vi "HWCEventHandler.vi"(8 "error in (no error)":errorcluster, 11 "HWController in":refnum<class "HWController.lvclass">) -> (0 "error out":errorcluster, 3 "HWController out":refnum<class "HWController.lvclass">)   [LabVIEW 2009, in "Hardware.lvlib" / "HWControllers.lvlib" / "HWController.lvclass"]
uses:
  HWController.lvclass
  HWController.lvclass/HWController.ctl
  HWControllerEvents/HWControllerEvents.lvclass
panel:
  out "configureTime":dbl
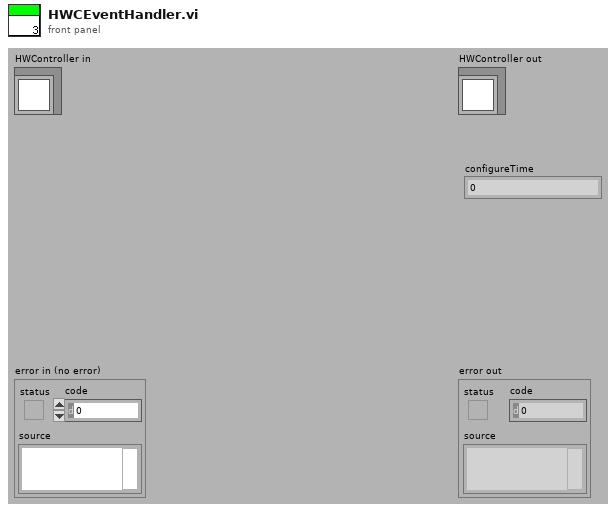
[diagram p1: front panel]
types:
  T1 = enum16{"Ready", "Compiling", "Configured", "Running", "Stopping", "Unresolved Error"}
  T2 = cluster{"incomingEventTypes":cluster{"start":cluster{"Boolean":bool}, "stop":cluster{"Boolean":bool}, "statusInquiry":cluster{"Boolean":bool}, "configure":cluster{"DPScriptPath":path, "TimeStamp":string, "HWLoop?":bool}, "resetError":cluster{"Boolean":bool}, "resourcesInquiry":cluster{"Boolean":bool}, "reserveResources":cluster{"HWList":string[]}, "initialise":cluster{"HWList":string[]}, "close":cluster{"Boolean":bool}, "resetAllChannels":cluster{"Boolean":bool}, "staticChannelUpdate":cluster{"channel_address":string, "calibratedValue":dbl}, "runScript":cluster{"DPScriptPath":path, "TimeStamp":string, "HWLoop?":bool}, "compilingScript":cluster{"Path":path}, "compiledScript":cluster{"Path":path, "timeCompileAt":string}, "compilerError":cluster{"Path":path}, "configureCompiledScript":cluster{"DPScriptPath":path, "TimeStamp":string, "HWLoop?":bool, "CompiledScript":cluster{"ScriptListCompiler.lvclass":refnum<class "ScriptListCompiler.lvclass">, "aoChannels":refnum<class "AnalogOutput.lvclass">[], "doChannels":refnum<class "DigitalOutput.lvclass">[], "rfChannels":refnum<class "DDSOutput.lvclass">[]}}, "restartCompiler":cluster{"restart":bool}, "staticRfChannelUpdate":cluster{"channel_address":string, "Output":cluster{"Frequency(MHz)":dbl, "Amplitude":dbl, "Phase":dbl, "OutputForm":enum16{"Sine", "Square", "Triangle", "Arbitrary"}}}}, "outgoingEventTypes":cluster{"HWStatus":cluster{"status":enum16{"Ready", "Compiling", "Configured", "Running", "Stopping", "Unresolved Error"}}, "error":cluster{"error out":errorcluster}, "resourcesAvailable":cluster{"availableHWList":string[], "reservedHWList":string[]}, "resourcesReserved":cluster{"reservedHWList":string[]}}}
  T3 = enum16{"start", "stop", "statusInquiry", "configure", "resetError", "resourcesInquiry", "reserveResources", "initialise", "resetAllChannels", "staticUpdate", "close", "HWStatus", "error", "resourcesAvailable", "resourcesReserved", "compilerError", "compiledScript", "compilingScript", "runScript", "configureCompiledScript", "restartCompiler", "staticRfChannelUpdate"}
  T4 = cluster{"start":cluster{"Boolean":bool}, "stop":cluster{"Boolean":bool}, "statusInquiry":cluster{"Boolean":bool}, "configure":cluster{"DPScriptPath":path, "TimeStamp":string, "HWLoop?":bool}, "resetError":cluster{"Boolean":bool}, "resourcesInquiry":cluster{"Boolean":bool}, "reserveResources":cluster{"HWList":string[]}, "initialise":cluster{"HWList":string[]}, "close":cluster{"Boolean":bool}, "resetAllChannels":cluster{"Boolean":bool}, "staticChannelUpdate":cluster{"channel_address":string, "calibratedValue":dbl}, "runScript":cluster{"DPScriptPath":path, "TimeStamp":string, "HWLoop?":bool}, "compilingScript":cluster{"Path":path}, "compiledScript":cluster{"Path":path, "timeCompileAt":string}, "compilerError":cluster{"Path":path}, "configureCompiledScript":cluster{"DPScriptPath":path, "TimeStamp":string, "HWLoop?":bool, "CompiledScript":cluster{"ScriptListCompiler.lvclass":refnum<class "ScriptListCompiler.lvclass">, "aoChannels":refnum<class "AnalogOutput.lvclass">[], "doChannels":refnum<class "DigitalOutput.lvclass">[], "rfChannels":refnum<class "DDSOutput.lvclass">[]}}, "restartCompiler":cluster{"restart":bool}, "staticRfChannelUpdate":cluster{"channel_address":string, "Output":cluster{"Frequency(MHz)":dbl, "Amplitude":dbl, "Phase":dbl, "OutputForm":enum16{"Sine", "Square", "Triangle", "Arbitrary"}}}}
  T5 = cluster{"DPScriptPath":path, "TimeStamp":string, "HWLoop?":bool}
  T6 = cluster{"DPScriptPath":path, "TimeStamp":string, "HWLoop?":bool, "CompiledScript":cluster{"ScriptListCompiler.lvclass":refnum<class "ScriptListCompiler.lvclass">, "aoChannels":refnum<class "AnalogOutput.lvclass">[], "doChannels":refnum<class "DigitalOutput.lvclass">[], "rfChannels":refnum<class "DDSOutput.lvclass">[]}}
  T7 = cluster{"ScriptListCompiler.lvclass":refnum<class "ScriptListCompiler.lvclass">, "aoChannels":refnum<class "AnalogOutput.lvclass">[], "doChannels":refnum<class "DigitalOutput.lvclass">[], "rfChannels":refnum<class "DDSOutput.lvclass">[]}
  T8 = cluster{"channel_address":string, "calibratedValue":dbl}
  T9 = cluster{"channel_address":string, "Output":cluster{"Frequency(MHz)":dbl, "Amplitude":dbl, "Phase":dbl, "OutputForm":enum16{"Sine", "Square", "Triangle", "Arbitrary"}}}
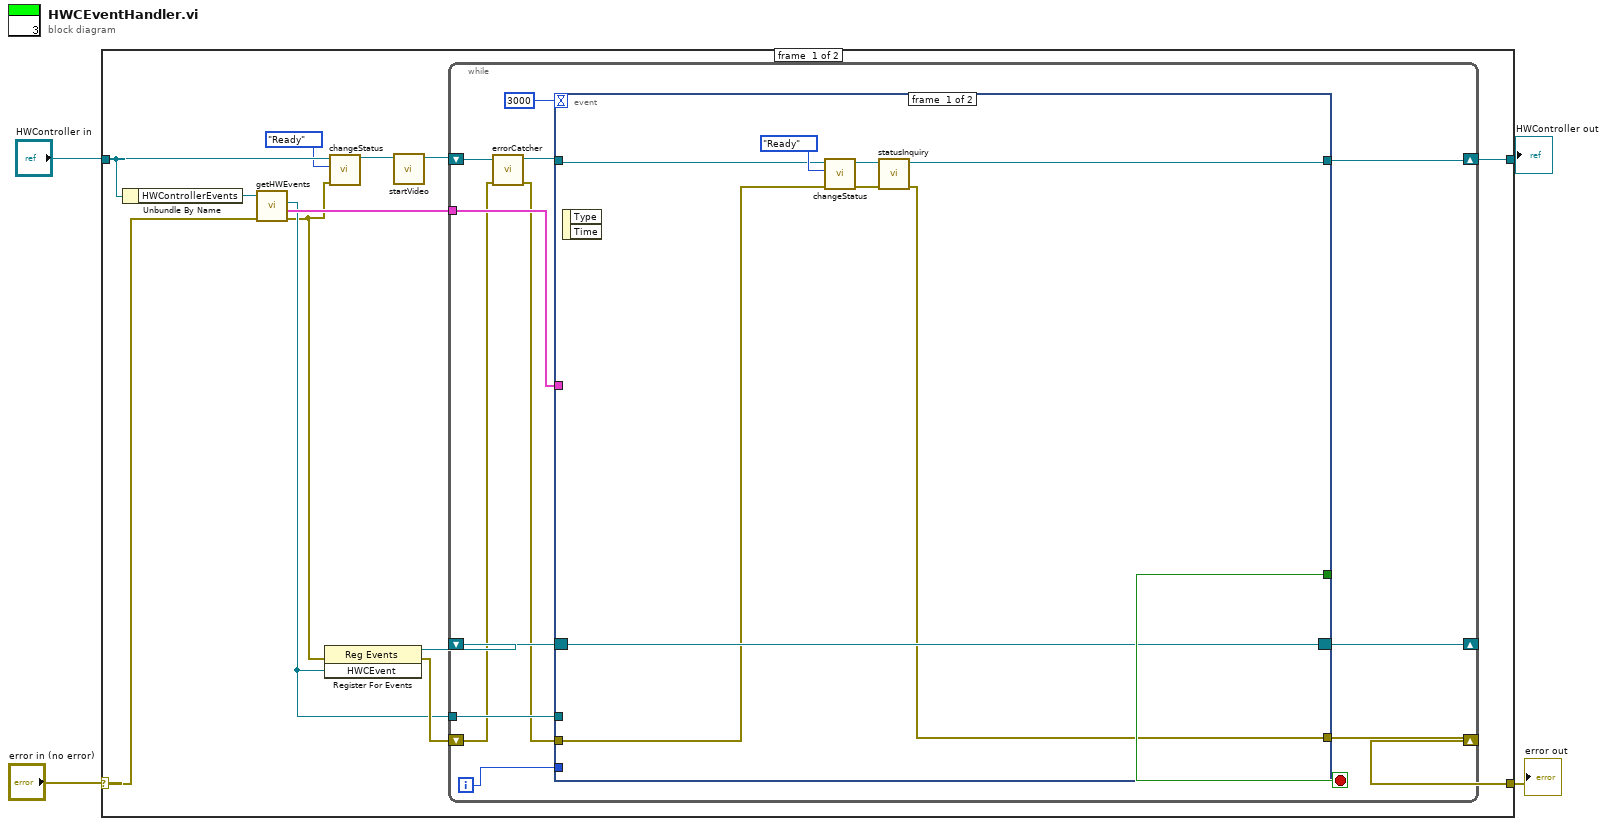
[diagram p0: block diagram]
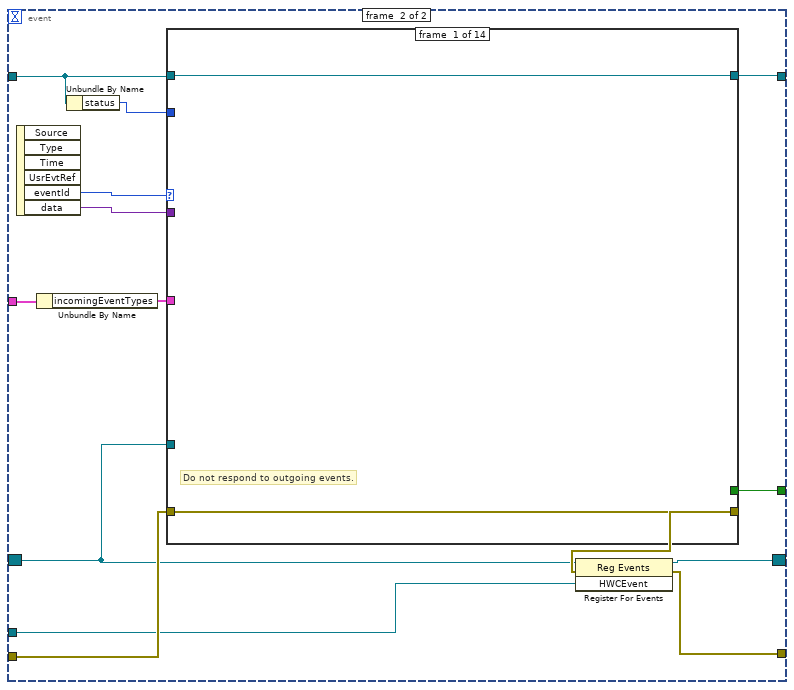
[diagram p2: hidden frame]
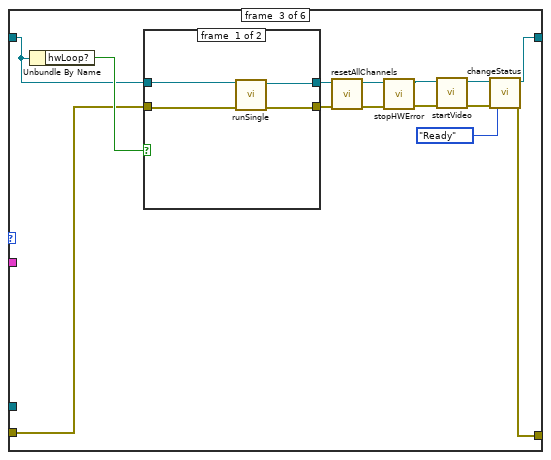
[diagram p5: hidden frame]
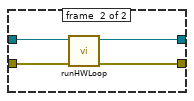
[diagram p6: hidden frame]
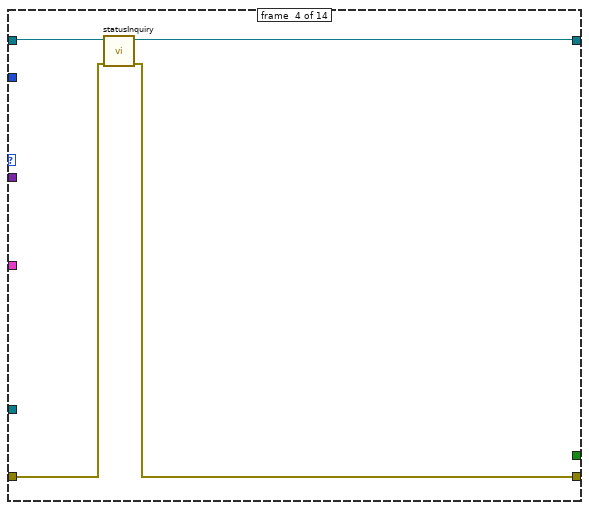
[diagram p11: hidden frame]
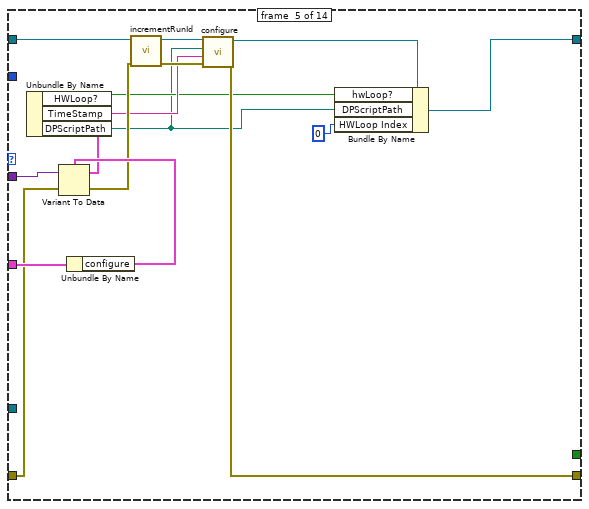
[diagram p12: hidden frame]
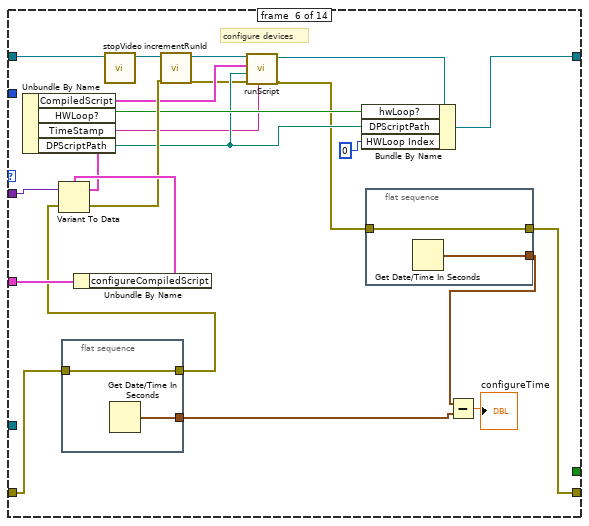
[diagram p13: hidden frame]
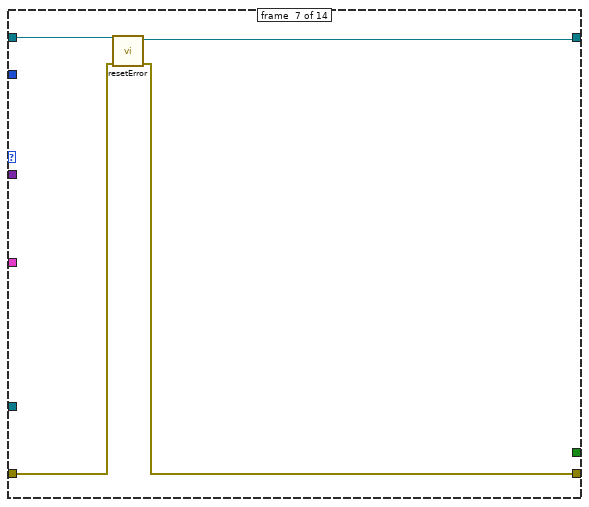
[diagram p14: hidden frame]
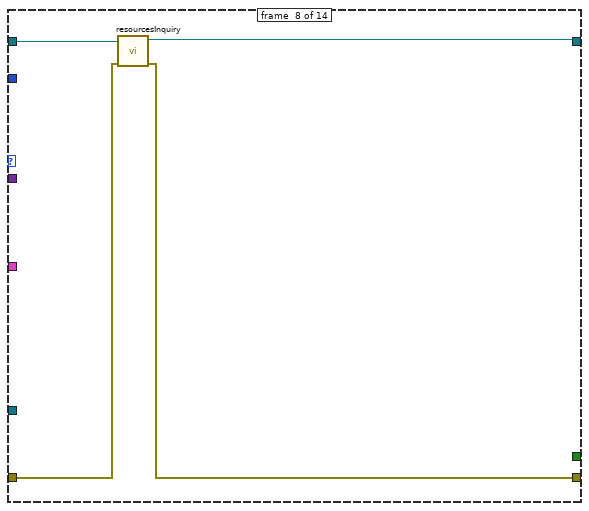
[diagram p15: hidden frame]
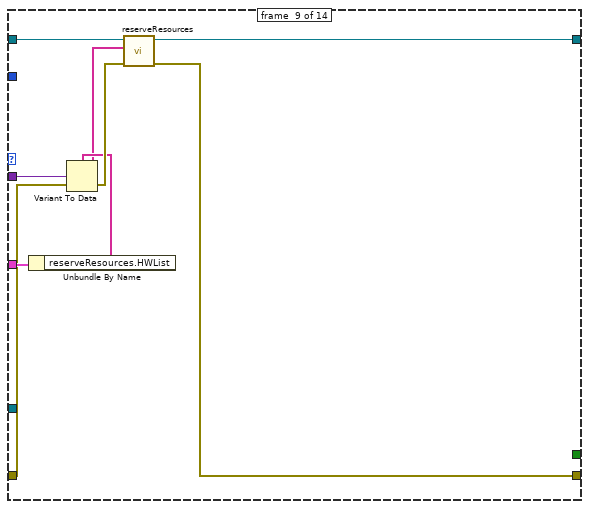
[diagram p16: hidden frame]
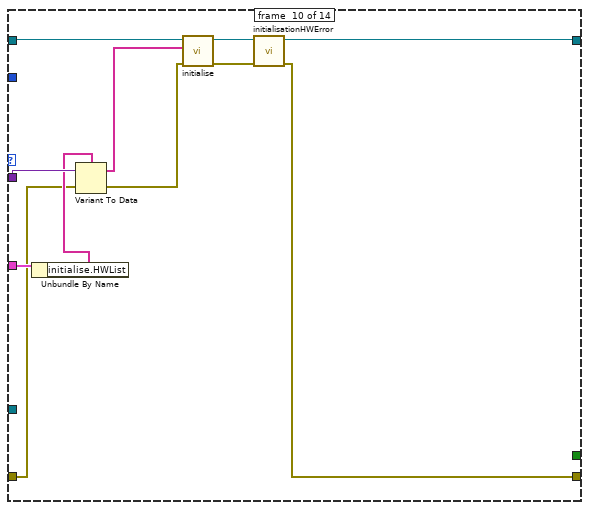
[diagram p17: hidden frame]
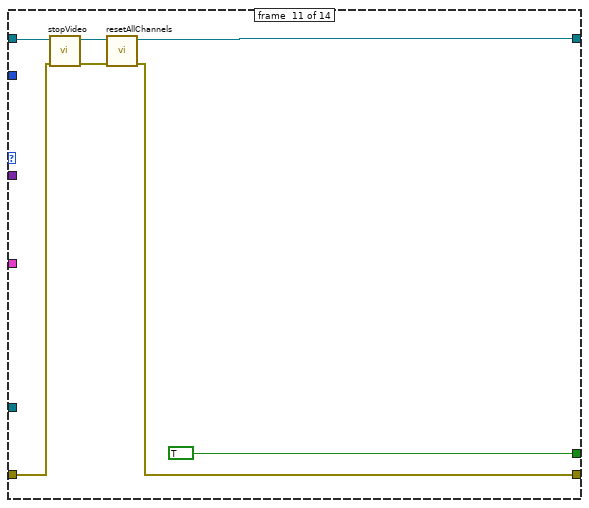
[diagram p18: hidden frame]
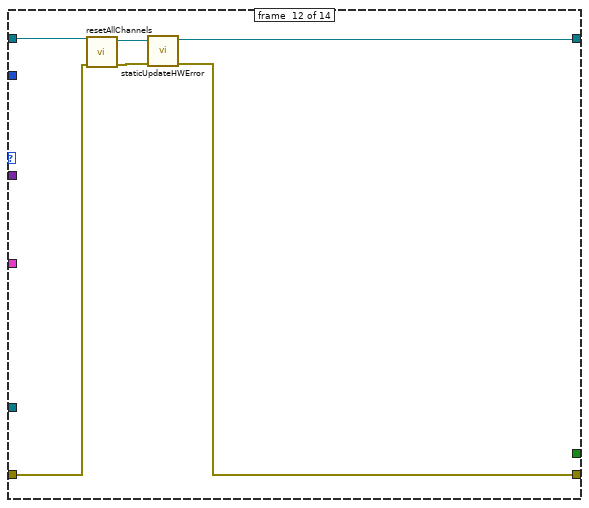
[diagram p19: hidden frame]
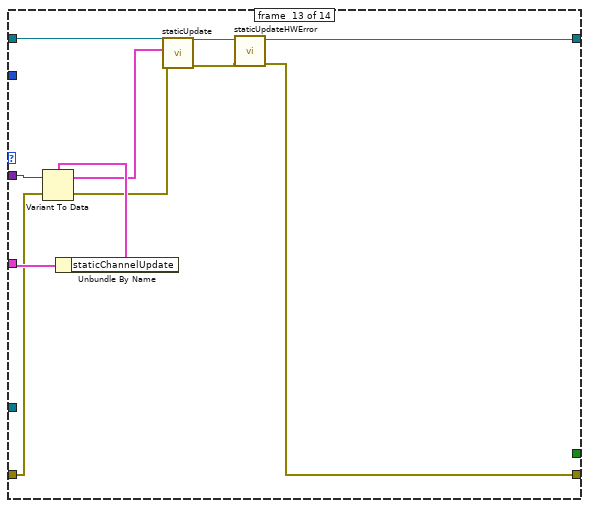
[diagram p20: hidden frame]
diagram:
  n1 = case shown="No Error" "error in (no error)" {
    selector: "error in (no error)" -> [w16 w207]
    tunnel: [w12 w207] -> w3
    tunnel: [w11 w206] -> w1
    tunnel: "HWController in" -> [w9 w206]
    frame #0 {
      n2 = Unbundle By Name(w9) -> ("HWControllerEvents"=w17:refnum<class "HWControllerEvents.lvclass">)
      n3 = call-dynamic "getHWEvents.vi"("error in (no error)"=w16, "HWControllerEvents in"=w17) -> ("error out"=w8:errorcluster, "eventDataTypes"=w13:T2, "HWCEvent"=w10:refnum<user-event>)  [unwired: 6 in, 1 out]
      n4 = register-events(error in=w8, w10) -> (reference out=w14:refnum<event-registration>, error out=w15:errorcluster)  [unwired: 1 in]
      n5 = call "changeStatus.vi"("error in (no error)"=w8, "status"=T1."Ready", "HWController in"=w9) -> ("HWController out"=w6:refnum<class "HWController.lvclass">)  [unwired: 7 in, 1 out]
      n6 = call-dynamic "startVideo.vi"("HWController in"=w6) -> ("HWController out"=w5:refnum<class "HWController.lvclass">)  [unwired: 9 in, 1 out]
      n7 = while {
        shift-right: [w30] -> w11
        shift-left: w5 -> [w22]
        shift-right: [w28] -> w12
        shift-left: w15 -> [w21]
        tunnel: w13 -> [w26]
        tunnel: w10 -> [w25]
        shift-right: [w24] -> _
        shift-left: w14 -> [w29]
        i -> [w18]
        stop <- w27 stop-if-true
        n8 = call-dynamic "errorCatcher.vi"("error in (no error)"=w21, "HWController in"=w22) -> ("error out"=w20:errorcluster, "HWController out"=w23:refnum<class "HWController.lvclass">)  [unwired: 8 in]
        n9 = event shown="[1] <HWCEvent>: User Event" {
          selector: w29 -> [w38 w44]
          dyn-events: [w38 w42] -> w24
          timeout: 3000 -> [_ _]
          tunnel: w23 -> [w33 w40]
          tunnel: [w37 w45] -> w30
          tunnel: [w36 w41] -> w28
          tunnel: w20 -> [w31 w51]
          tunnel: [_ w50] -> w27
          tunnel: w26 -> [_ w49]
          tunnel: w25 -> [_ w43]
          tunnel: w18 -> [_ _]
          event #0 {
            n10 = event-data() -> ()  [unwired: 1 in, 2 out]
            n11 = call "changeStatus.vi"("error in (no error)"=w31, "status"=T1."Ready", "HWController in"=w33) -> ("error out"=w32:errorcluster, "HWController out"=w34:refnum<class "HWController.lvclass">)  [unwired: 7 in]
            n12 = call-dynamic "statusInquiry.vi"("error in (no error)"=w32, "HWController in"=w34) -> ("error out"=w36:errorcluster, "HWController out"=w37:refnum<class "HWController.lvclass">)  [unwired: 8 in]
          }
          event #1 {
            n13 = event-data() -> ("eventId"=w52:T3, "data"=w47:variant)  [unwired: 1 in, 4 out]
            n14 = Unbundle By Name(w49) -> ("incomingEventTypes"=w48:T4)
            n15 = Unbundle By Name(w40) -> ("status"=w39:T1)
            n16 = case shown="\"start\"" w52 {
              tunnel: w40 -> [w54 w61 w95 w99 w109 w117 w146 w150 w158 w169 w174 w183 w194 w201]
              tunnel: [w54 w59 w95 w98 w101 w132 w145 w149 w157 w160 w176 w179 w185 w195] -> w45
              tunnel: w51 -> [w53 w57 w94 w97 w112 w124 w144 w148 w154 w165 w171 w182 w189 w202]
              tunnel: [w53 w58 w94 w96 w110 w121 w143 w147 w156 w161 w175 w178 w184 w196] -> w46
              tunnel: [_ _ _ _ _ _ _ _ _ _ TRUE _ _ _] -> w50
              tunnel: w48 -> [_ w55 _ _ w115 w138 _ _ w159 w170 _ _ w192 w204]
              tunnel: w47 -> [_ _ _ _ w113 w136 _ _ w155 w168 _ _ w193 w205]
              tunnel: w44 -> [_ w60 _ _ _ _ _ _ _ _ _ _ _ _]
              tunnel: w39 -> [_ w56 _ _ _ _ _ _ _ _ _ _ _ _]
              frame #0 {
                # "Do not respond to outgoing events."
              }
              frame #1 {
                n17 = case shown="\"Configured\"" w56 {
                  tunnel: w61 -> [w63 w65 w76 w89 w91 w93]
                  tunnel: w60 -> [_ _ _ _ _ _]
                  tunnel: [w63 w65 w66 w89 w91 w93] -> w59
                  tunnel: [w62 w64 w72 w88 w90 w92] -> w58
                  tunnel: w57 -> [w62 w64 w73 w88 w90 w92]
                  tunnel: w55 -> [_ _ _ _ _ _]
                  frame #0 {
                  }
                  frame #1 {
                  }
                  frame #2 {
                    n18 = Unbundle By Name(w76) -> ("hwLoop?"=w79:bool)
                    n19 = case shown="True" w79 {
                      tunnel: w73 -> [w82 w84]
                      tunnel: [w81 w86] -> w78
                      tunnel: [w80 w85] -> w77
                      tunnel: w76 -> [w83 w87]
                      frame #0 {
                        n20 = call "runSingle.vi"("error in (no error)"=w82, "HWController in"=w83) -> ("error out"=w80:errorcluster, "HWController out"=w81:refnum<class "HWController.lvclass">)  [unwired: 6 in, 2 out]
                      }
                      frame #1 {
                        n21 = call "runHWLoop.vi"("error in (no error)"=w84, "HWController in"=w87) -> ("error out"=w85:errorcluster, "HWController out"=w86:refnum<class "HWController.lvclass">)  [unwired: 8 in]
                      }
                    }
                    n22 = call-dynamic "resetAllChannels.vi"("error in (no error)"=w77, "HWController in"=w78) -> ("error out"=w74:errorcluster, "HWController out"=w75:refnum<class "HWController.lvclass">)  [unwired: 8 in]
                    n23 = call-dynamic "stopHWError.vi"("error in (no error)"=w74, "HWController in"=w75) -> ("error out"=w69:errorcluster, "HWController out"=w70:refnum<class "HWController.lvclass">)  [unwired: 8 in]
                    n24 = call-dynamic "startVideo.vi"("error in (no error)"=w69, "HWController in"=w70) -> ("error out"=w67:errorcluster, "HWController out"=w68:refnum<class "HWController.lvclass">)  [unwired: 8 in]
                    n25 = call "changeStatus.vi"("error in (no error)"=w67, "status"=T1."Ready", "HWController in"=w68) -> ("error out"=w72:errorcluster, "HWController out"=w66:refnum<class "HWController.lvclass">)  [unwired: 7 in]
                  }
                  frame #3 {
                  }
                  frame #4 {
                  }
                  frame #5 {
                  }
                }
              }
              frame #2 {
              }
              frame #3 {
                n26 = call-dynamic "statusInquiry.vi"("error in (no error)"=w97, "HWController in"=w99) -> ("error out"=w96:errorcluster, "HWController out"=w98:refnum<class "HWController.lvclass">)  [unwired: 8 in]
              }
              frame #4 {
                n27 = Unbundle By Name(w115) -> ("configure"=w114:T5)
                n28 = Variant To Data(error in=w112, Variant=w113, type=w114) -> (error out=w107:errorcluster, data=w111:T5)
                n29 = Unbundle By Name(w111) -> ("HWLoop?"=w104:bool, "TimeStamp"=w105:string, "DPScriptPath"=w102:path)
                n30 = call "incrementRunId.vi"("error in (no error)"=w107, "HWController in"=w109) -> ("error out"=w106:errorcluster, "HWController out"=w108:refnum<class "HWController.lvclass">)  [unwired: 8 in]
                n31 = call-dynamic "configure.vi"("error in (no error)"=w106, "timeStamp"=w105, "Path"=w102, "HWController in"=w108) -> ("error out"=w110:errorcluster, "HWController out"=w103:refnum<class "HWController.lvclass">)  [unwired: 6 in]
                n32 = Bundle By Name(cluster=w103, "hwLoop?"=w104, "DPScriptPath"=w102, "HWLoop Index"=0) -> (w101:refnum<class "HWController.lvclass">)
              }
              frame #5 {
                # "configure devices"
                n33 = flat-sequence {
                  tunnel: w124 -> [w142]
                  tunnel: [w142] -> w123
                  tunnel: [w141] -> w120
                  frame #0 {
                    n34 = Get Date/Time In Seconds() -> (seconds since 1Jan1904=w141:timestamp)
                  }
                }
                n35 = Unbundle By Name(w138) -> ("configureCompiledScript"=w137:T6)
                n36 = Variant To Data(error in=w123, Variant=w136, type=w137) -> (error out=w134:errorcluster, data=w135:T6)
                n37 = Unbundle By Name(w135) -> ("CompiledScript"=w129:T7, "HWLoop?"=w133:bool, "TimeStamp"=w127:string, "DPScriptPath"=w128:path)
                n38 = call-dynamic "stopVideo.vi"("HWController in"=w117) -> ("HWController out"=w116:refnum<class "HWController.lvclass">)  [unwired: 9 in, 1 out]
                n39 = call "incrementRunId.vi"("error in (no error)"=w134, "HWController in"=w116) -> ("error out"=w126:errorcluster, "HWController out"=w130:refnum<class "HWController.lvclass">)  [unwired: 8 in]
                n40 = call-dynamic "runScript.vi"("timeStamp"=w127, "error in (no error)"=w126, "Path"=w128, "CompiledScript"=w129, "HWController in"=w130) -> ("error out"=w122:errorcluster, "HWController out"=w125:refnum<class "HWController.lvclass">)  [unwired: 5 in]
                n41 = Bundle By Name(cluster=w125, "hwLoop?"=w133, "DPScriptPath"=w128, "HWLoop Index"=0) -> (w132:refnum<class "HWController.lvclass">)
                n42 = flat-sequence {
                  tunnel: w122 -> [w140]
                  tunnel: [w140] -> w121
                  tunnel: [w139] -> w119
                  frame #0 {
                    n43 = Get Date/Time In Seconds() -> (seconds since 1Jan1904=w139:timestamp)
                  }
                }
                n44 = Subtract(x=w119, y=w120) -> (x-y=→"configureTime":dbl)
              }
              frame #6 {
                n45 = call-dynamic "resetError.vi"("error in (no error)"=w144, "HWController in"=w146) -> ("error out"=w143:errorcluster, "HWController out"=w145:refnum<class "HWController.lvclass">)  [unwired: 8 in]
              }
              frame #7 {
                n46 = call-dynamic "resourcesInquiry.vi"("error in (no error)"=w148, "HWController in"=w150) -> ("error out"=w147:errorcluster, "HWController out"=w149:refnum<class "HWController.lvclass">)  [unwired: 8 in]
              }
              frame #8 {
                n47 = Unbundle By Name(w159) -> ("reserveResources.HWList"=w152:string[])
                n48 = Variant To Data(error in=w154, Variant=w155, type=w152) -> (error out=w153:errorcluster, data=w151:string[])
                n49 = call-dynamic "reserveResources.vi"("error in (no error)"=w153, "HWList"=w151, "HWController in"=w158) -> ("error out"=w156:errorcluster, "HWController out"=w157:refnum<class "HWController.lvclass">)  [unwired: 7 in]
              }
              frame #9 {
                n50 = Unbundle By Name(w170) -> ("initialise.HWList"=w167:string[])
                n51 = Variant To Data(error in=w165, Variant=w168, type=w167) -> (error out=w164:errorcluster, data=w166:string[])
                n52 = call-dynamic "initialise.vi"("error in (no error)"=w164, "HWList"=w166, "HWController in"=w169) -> ("error out"=w162:errorcluster, "HWController out"=w163:refnum<class "HWController.lvclass">)  [unwired: 7 in]
                n53 = call-dynamic "initialisationHWError.vi"("error in (no error)"=w162, "HWController in"=w163) -> ("error out"=w161:errorcluster, "HWController out"=w160:refnum<class "HWController.lvclass">)  [unwired: 8 in]
              }
              frame #10 {
                n54 = call-dynamic "stopVideo.vi"("error in (no error)"=w171, "HWController in"=w174) -> ("error out"=w172:errorcluster, "HWController out"=w173:refnum<class "HWController.lvclass">)  [unwired: 8 in]
                n55 = call-dynamic "resetAllChannels.vi"("error in (no error)"=w172, "HWController in"=w173) -> ("error out"=w175:errorcluster, "HWController out"=w176:refnum<class "HWController.lvclass">)  [unwired: 8 in]
              }
              frame #11 {
                n56 = call-dynamic "resetAllChannels.vi"("error in (no error)"=w182, "HWController in"=w183) -> ("error out"=w180:errorcluster, "HWController out"=w181:refnum<class "HWController.lvclass">)  [unwired: 8 in]
                n57 = call-dynamic "staticUpdateHWError.vi"("error in (no error)"=w180, "HWController in"=w181) -> ("error out"=w178:errorcluster, "HWController out"=w179:refnum<class "HWController.lvclass">)  [unwired: 8 in]
              }
              frame #12 {
                n58 = Unbundle By Name(w192) -> ("staticChannelUpdate"=w191:T8)
                n59 = Variant To Data(error in=w189, Variant=w193, type=w191) -> (error out=w188:errorcluster, data=w190:T8)
                n60 = call-dynamic "staticUpdate.vi"("error in (no error)"=w188, "staticChannelUpdate"=w190, "HWController in"=w194) -> ("error out"=w186:errorcluster, "HWController out"=w187:refnum<class "HWController.lvclass">)  [unwired: 7 in]
                n61 = call-dynamic "staticUpdateHWError.vi"("error in (no error)"=w186, "HWController in"=w187) -> ("error out"=w184:errorcluster, "HWController out"=w185:refnum<class "HWController.lvclass">)  [unwired: 8 in]
              }
              frame #13 {
                n62 = Unbundle By Name(w204) -> ("staticRfChannelUpdate"=w203:T9)
                n63 = Variant To Data(error in=w202, Variant=w205, type=w203) -> (error out=w199:errorcluster, data=w200:T9)
                n64 = call-dynamic "staticRFChannelUpdate.vi"("error in (no error)"=w199, "staticChannelUpdate"=w200, "HWController in"=w201) -> ("error out"=w197:errorcluster, "HWController out"=w198:refnum<class "HWController.lvclass">)  [unwired: 7 in]
                n65 = call-dynamic "staticUpdateHWError.vi"("error in (no error)"=w197, "HWController in"=w198) -> ("error out"=w196:errorcluster, "HWController out"=w195:refnum<class "HWController.lvclass">)  [unwired: 8 in]
              }
            }
            n66 = register-events(reference=w44, error in=w46, w43) -> (reference out=w42:refnum<event-registration>, error out=w41:errorcluster)
          }
        }
      }
    }
    frame #1 {
    }
  }
  "error out" <- w3
  "HWController out" <- w1
